vi "send.status.vi"(6 "iteration":i32, 8 "error in (no error)":errorcluster, 11 "comic_crawler in":refnum<class "comic_crawler.lvclass">) -> (0 "error out":errorcluster, 2 "status":T1, 3 "comic_crawler out":refnum<class "comic_crawler.lvclass">)   [LabVIEW 2024, in "comic_crawler.lvclass"]
uses:
  comic_crawler.lvclass
  status--cluster.ctl
  comic_crawler.lvclass/comic_crawler.ctl
  1d6cef87-03dc-4078-b754-2ad5cfa3a6d1.vi
  <userlib>/_MGI/1D Array/MGI Running Average/MGI Running Average(DBL).vi
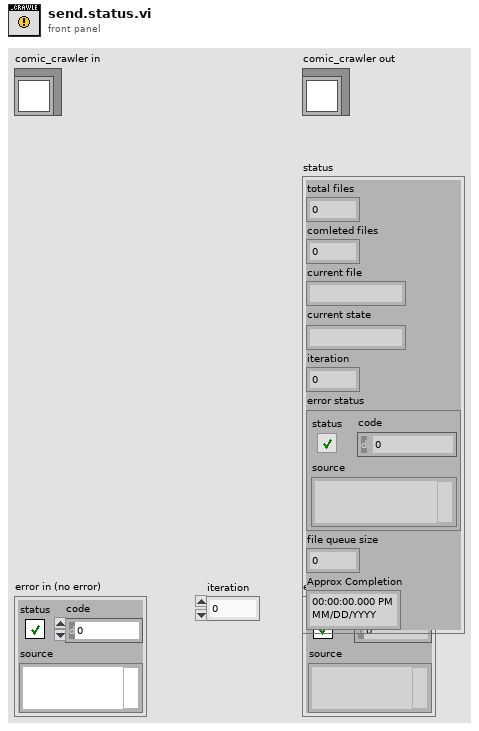
[diagram p1: front panel]
types:
  T1 = typedef "comic_crawler.lvclass/status--cluster.ctl" = cluster{"total files":i32, "comleted files":i32, "current file":string, "current state":string, "iteration":i32, "error status":errorcluster, "file queue size":i32, "Approx Completion":timestamp}
  T2 = typedef "comic_crawler.lvclass/daemon.states--enum.ctl" = enum16{"start search", "idle", "set timer", "running", "stop search", "wait", "set delay", "shut down"}
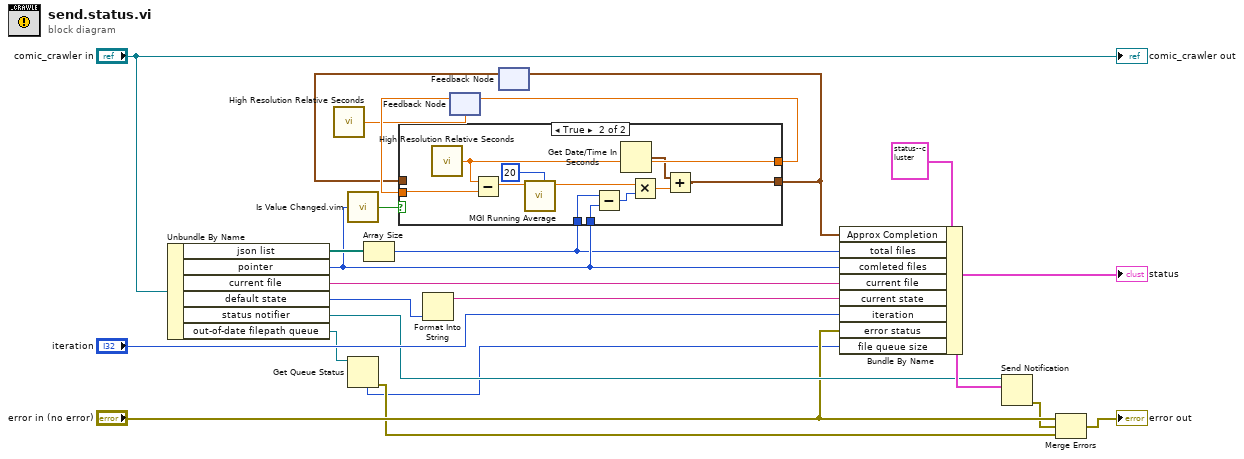
[diagram p0: block diagram]
diagram:
  n1 = Unbundle By Name("comic_crawler in") -> ("json list"=w10:path[], "pointer"=w4:i32, "current file"=w19:string, "default state"=w17:T2, "status notifier"=w16:refnum<notifier>, "out-of-date filepath queue"=w12:refnum<queue>)
  n2 = call <vilib>:"High Resolution Relative Seconds.vi"() -> ("relative seconds"=w6:dbl)
  n3 = call "Is Value Changed.vim"("value"=w4) -> ("changed or first call?"=w9:bool)
  n4 = Get Queue Status(queue=w12) -> (error out=w11:errorcluster, # elements in queue=w5:i32)  [unwired: 2 in, 6 out]
  n5 = Array Size(array=w10) -> (size(s)=w3:i32)
  n6 = Format Into String(w17) -> (resulting string=w18:string)  [unwired: 3 in, 1 out]
  n7 = feedback #1(w6) -> (w7:dbl)
  n8 = feedback #2() -> (w1:timestamp)  [unwired: 1 in]
  n9 = case shown="True" w9 {
    tunnel: [w25 w28] -> w8
    tunnel: w7 -> [w25 w36]
    tunnel: w4 -> [_ w31]
    tunnel: w3 -> [_ w30]
    tunnel: [w24 w26] -> w2
    tunnel: w1 -> [w24 _]
    frame False {
    }
    frame True {
      n10 = call <vilib>:"High Resolution Relative Seconds.vi"() -> ("relative seconds"=w28:dbl)
      n11 = Subtract(x=w28, y=w36) -> (x-y=w35:dbl)
      n12 = call-poly <userlib>:"MGI Running Average.vi"("Averaging Size"=20, "Value"=w35) -> ("Average"=w33:dbl)  [unwired: 9 in]
      n13 = Subtract(x=w30, y=w31) -> (x-y=w32:i32)
      n14 = Get Date/Time In Seconds() -> (seconds since 1Jan1904=w27:timestamp)
      n15 = Multiply(x=w33, y=w32) -> (x*y=w29:dbl)
      n16 = Add(x=w27, y=w29) -> (x+y=w26:timestamp)
    }
  }
  n17 = feedback-in #1(w8) -> ()
  n18 = feedback-in #2(w2) -> ()
  n19 = Bundle By Name(cluster=T1 {"total files"=0, "comleted files"=0, "current file"="", "current state"="", "iteration"=0, "error status"={"status"=FALSE, "code"=0, "source"=""}, "file queue size"=0, "Approx Completion"=timestamp(0 s since 1904-01-01)} ("status"), "Approx Completion"=w2, "total files"=w3, "comleted files"=w4, "current file"=w19, "current state"=w18, "iteration"="iteration", "error status"="error in (no error)", "file queue size"=w5) -> (w22:T1)
  "status" <- w22
  n20 = Send Notification(notification=w22, notifier=w16) -> (error out=w14:errorcluster)  [unwired: 1 in, 1 out]
  n21 = Merge Errors("error in (no error)", w14, w11) -> (→"error out":errorcluster)
  "comic_crawler out" <- "comic_crawler in"
